vi "BRig_RT__Case_Exp__State_endTrial__v10.vi"(6 "input_dataBlock":u16[][](array[numeric]), 9 "input_timeStamp_start":dbl, 10 "input_dataTrial":u16[][](array[numeric]), 11 "input_dataCurrent":u16[](array[numeric])) -> (0 "output_BTPRavg":dbl, 1 "output_T2Ravg":dbl, 2 "output_dataTrial":u16[][](array[numeric]), 3 "output_dataCurrent":u16[](array[numeric]), 4 "output_R(F)_or_L(T)":bool, 5 "output_runTime":dbl)   [LabVIEW 2014]
panel:
  in  "input_dataExp":u16[](array[numeric])
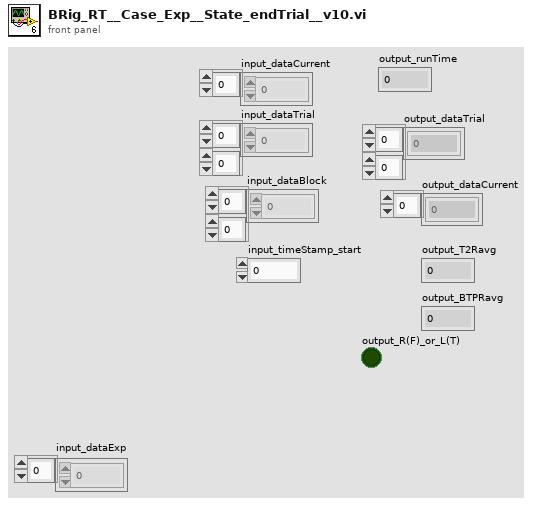
[diagram p1: front panel]
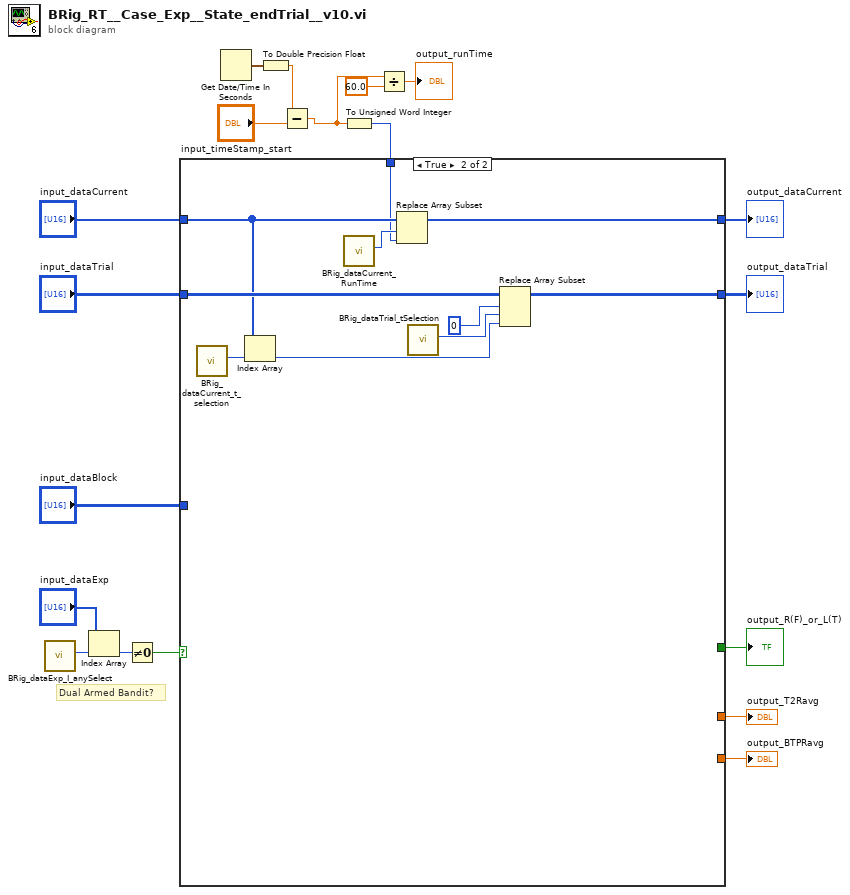
[diagram p0: block diagram]
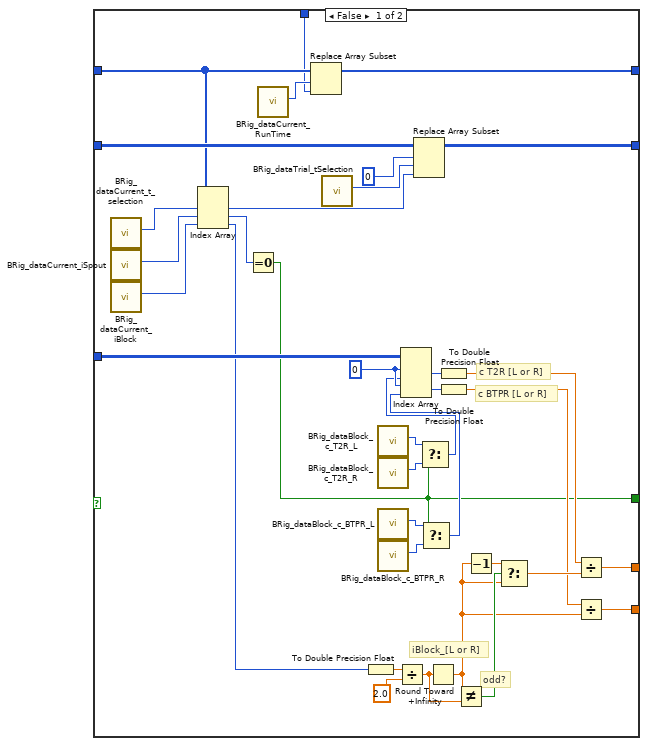
[diagram p2: hidden frame]
diagram:
  # "Dual Armed Bandit?"
  n1 = call "BRig_dataExp_I_anySelect.vi"() -> ("output_I_anySelect"=w4:i32)  [unwired: 11 in]
  n2 = Index Array(array="input_dataExp", index=w4) -> (element=w3:u16)
  n3 = Not Equal To 0?(x=w3) -> (x != 0?=w1:bool)
  n4 = Get Date/Time In Seconds() -> (seconds since 1Jan1904=w16:timestamp)
  n5 = To Double Precision Float(number=w16) -> (double precision float=w14:dbl)
  n6 = Subtract(x=w14, y="input_timeStamp_start") -> (x-y=w11:dbl)
  n7 = To Unsigned Word Integer(number=w11) -> (unsigned 16bit integer=w13:u16)
  n8 = case shown="True" w1 {
    tunnel: "input_dataTrial" -> [w54 w64]
    tunnel: [w53 w63] -> w18
    tunnel: "input_dataCurrent" -> [w52 w62]
    tunnel: w13 -> [w50 w60]
    tunnel: [w49 w59] -> w12
    tunnel: "input_dataBlock" -> [w42 _]
    tunnel: [w39 _] -> w7
    tunnel: [w38 _] -> w6
    tunnel: [w20 _] -> w5
    frame False {
      w41 = 0
      # "c BTPR [L or R]"
      # "c T2R [L or R]"
      # "odd?"
      # "iBlock_[L or R]"
      n9 = call "BRig_dataCurrent_t_selection.vi"() -> ("output_t_selection"=w47:i32)  [unwired: 11 in]
      n10 = call "BRig_dataCurrent_iSpout.vi"() -> ("output_iSpout"=w45:i32)  [unwired: 11 in]
      n11 = call "BRig_dataCurrent_iBlock.vi"() -> ("output_iBlock"=w43:i32)  [unwired: 11 in]
      n12 = Index Array(array=w52, index #1=w47, index #2=w45, index #3=w43) -> (element #1=w46:u16, element #2=w44:u16, element #3=w40:u16)
      n13 = Equal To 0?(x=w44) -> (x = 0?=w20:bool)
      n14 = call "BRig_dataCurrent_RunTime.vi"() -> ("output_RunTime"=w51:i32)  [unwired: 11 in]
      n15 = Replace Array Subset(array=w52, new element=w50, index=w51) -> (w49:u16[])
      n16 = call "BRig_dataTrial_tSelection.vi"() -> ("output_tSelection"=w55:i32)  [unwired: 11 in]
      n17 = To Double Precision Float(number=w40) -> (double precision float=w31:dbl)
      n18 = call "BRig_dataBlock_c_T2R_L.vi"() -> ("output_c_T2R_L"=w36:i32)  [unwired: 11 in]
      n19 = call "BRig_dataBlock_c_T2R_R.vi"() -> ("output_c_T2R_R"=w37:i32)  [unwired: 11 in]
      n20 = call "BRig_dataBlock_c_BTPR_L.vi"() -> ("output_c_BTPR_L"=w34:i32)  [unwired: 11 in]
      n21 = call "BRig_dataBlock_c_BTPR_R.vi"() -> ("output_c_BTPR_R"=w35:i32)  [unwired: 11 in]
      n22 = Divide(x=w31, y=2.0) -> (x/y=w29:dbl)
      n23 = Replace Array Subset(array=w54, new element=w46, index (row)=0, index (col)=w55) -> (w53:u16[][])
      n24 = Select(t=w36, s=w20, f=w37) -> (s? t:f=w33:i32)
      n25 = Select(t=w34, s=w20, f=w35) -> (s? t:f=w32:i32)
      n26 = Index Array(array=w42, index (row) #1=w41, index (col) #1=w33, index (row) #2=w41, index (col) #2=w32) -> (element #1=w24:u16, element #2=w25:u16)
      n27 = Round Toward +Infinity(x=w29) -> (ceil(x): smallest int >= x=w23:dbl)
      n28 = To Double Precision Float(number=w24) -> (double precision float=w22:dbl)
      n29 = To Double Precision Float(number=w25) -> (double precision float=w21:dbl)
      n30 = Not Equal?(x=w23, y=w29) -> (x != y?=w27:bool)
      n31 = Decrement(x=w23) -> (x-1=w28:dbl)
      n32 = Select(t=w28, s=w27, f=w23) -> (s? t:f=w26:dbl)
      n33 = Divide(x=w22, y=w26) -> (x/y=w39:dbl)
      n34 = Divide(x=w21, y=w23) -> (x/y=w38:dbl)
    }
    frame True {
      n35 = call "BRig_dataCurrent_t_selection.vi"() -> ("output_t_selection"=w57:i32)  [unwired: 11 in]
      n36 = Index Array(array=w62, index=w57) -> (element=w56:u16)
      n37 = call "BRig_dataCurrent_RunTime.vi"() -> ("output_RunTime"=w61:i32)  [unwired: 11 in]
      n38 = Replace Array Subset(array=w62, new element=w60, index=w61) -> (w59:u16[])
      n39 = call "BRig_dataTrial_tSelection.vi"() -> ("output_tSelection"=w65:i32)  [unwired: 11 in]
      n40 = Replace Array Subset(array=w64, new element=w56, index (row)=0, index (col)=w65) -> (w63:u16[][])
    }
  }
  "output_dataTrial" <- w18
  "output_dataCurrent" <- w12
  "output_T2Ravg" <- w7
  "output_BTPRavg" <- w6
  "output_R(F)_or_L(T)" <- w5
  n41 = Divide(x=w11, y=60.0) -> (x/y=→"output_runTime":dbl)
